vi "扫描测试数据保存.vi"(8 "错误输入（无错误）":errorcluster, 10 "扫描数据":dbl[][](array[numeric]), 11 "start path":path=path "D:/Data") -> (0 "错误输出":errorcluster, 3 "路径":path)   [LabVIEW 2020]
uses:
  <vilib>/Utility/file.llb/Write Delimited Spreadsheet (DBL).vi
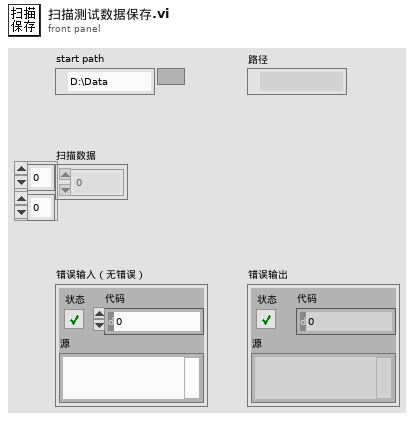
[diagram p1: front panel]
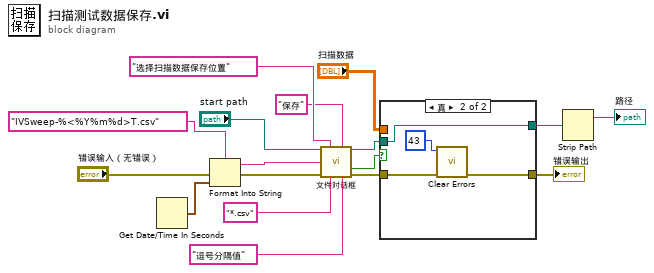
[diagram p0: block diagram]
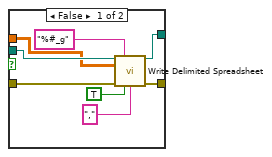
[diagram p2: hidden frame]
diagram:
  n1 = Get Date/Time In Seconds() -> (seconds since 1Jan1904=w5:timestamp)
  n2 = Format Into String(format string="IVSweep-%<%Y%m%d>T.csv" ("格式字符串"), error in="错误输入（无错误）", w5) -> (resulting string=w7:string, error out=w6:errorcluster)  [unwired: 1 in]
  n3 = call "文件对话框"("start path"="start path", "prompt"="选择扫描数据保存位置", "button label"="保存", "default name"=w7, "error in"=w6, "pattern (all files)"="*.csv", "pattern label"="逗号分隔值") -> ("selected path"=w15:path, "cancelled"=w17:bool, "error out"=w12:errorcluster)  [unwired: 5 in, 1 out]
  n4 = case shown="真" w17 {
    tunnel: w12 -> [w25 w29]
    tunnel: [w24 w28] -> w14
    tunnel: w15 -> [w23 w26]
    tunnel: "扫描数据" -> [w22 _]
    tunnel: [w18 w26] -> w2
    frame False {
      n5 = call-poly <vilib>:"Write Delimited Spreadsheet.vi"("file path (dialog if empty)"=w23, "format (%.3f)"="%#_g", "2D data"=w22, "error in (no error)"=w25, "transpose? (no:F)"=TRUE, "delimiter (\\t)"="," ("delimiter (\\t)")) -> ("new file path (Not A Path if cancelled)"=w18:path, "error out"=w24:errorcluster)  [unwired: 8 in]
    }
    frame True {
      n6 = call <vilib>:"Clear Errors.vi"("error in (no error)"=w29, "specific error code to clear (0: all)"=43) -> ("error out"=w28:errorcluster)  [unwired: 4 in, 1 out]
    }
  }
  "错误输出" <- w14
  n7 = Strip Path(path=w2) -> (stripped path=→"路径":path)  [unwired: 1 out]
